vi "acquisition test fixed exposure 6.vi"() -> ()   [LabVIEW 2023]
uses:
  <vilib>/userDefined/High Color/IMAQdx.ctl
  <vilib>/vision/driver/IMAQdx.llb/IMAQdx Acquisition Mode.ctl
  <vilib>/vision/Avi.llb/IMAQ AVI2 Refnum.ctl
  <vilib>/vision/Image Controls.llb/IMAQ Image.ctl
  <vilib>/vision/driver/IMAQdx.llb/IMAQdx Buffer Number Mode.ctl
  <vilib>/DAQmx/write.llb/DAQmx Write (Analog 1D Wfm NChan NSamp).vi
  <vilib>/DAQmx/read.llb/DAQmx Read (Analog 1D Wfm NChan NSamp).vi
  <extravilib>/ChannelInstances/Tag-bool/Read With Abort.vi
  <vilib>/Utility/High Resolution Relative Seconds.vi
  <extravilib>/ChannelInstances/Tag-bool/Write With Abort.vi
  <vilib>/DAQmx/create/channels.llb/DAQmx Create Channel (AI-Voltage-Basic).vi
  <vilib>/DAQmx/configure/timing.llb/DAQmx Timing (Sample Clock).vi
  <vilib>/DAQmx/create/channels.llb/DAQmx Create Channel (AO-Voltage-Basic).vi
  <vilib>/DAQmx/configure/trigger.llb/DAQmx Start Trigger (Digital Edge).vi
  <vilib>/DAQmx/miscellaneous.llb/DAQmx Fill In Error Info.vi
  <extravilib>/ChannelInstances/Tag-bool/Instantiate.vi
  <extravilib>/ChannelInstances/Tag-bool/EndpointRead.vi
  <vilib>/vision/EDVR.llb/IMAQ ImageToEDVR.vi
  <vilib>/vision/EDVR.llb/IMAQ ImageToEDVR 1D U8.vi
  <vilib>/vision/EDVR.llb/IMAQ ImageToEDVR 1D I16.vi
  <vilib>/vision/EDVR.llb/IMAQ ImageToEDVR 1D U32.vi
  <vilib>/vision/EDVR.llb/IMAQ ImageToEDVR 1D U16.vi
  <vilib>/Utility/file.llb/Write Delimited Spreadsheet (string).vi
  <extravilib>/ChannelInstances/Tag-bool/Endpoint.vi
  <vilib>/Waveform/WDTOps.llb/WDT Append Waveforms DBL.vi
  <extravilib>/ChannelInstances/Tag-bool.lvlib
  <vilib>/vision/driver/NI_Vision_Acquisition_Software.lvlib
  <resource>/objmgr/imaqdx.rc
  <vilib>/measure/NI_MABase.lvlib
  <resource>/objmgr/daqmx.rc
panel:
  out "Image Display":T1(plugin-control)
  out "SampClk.Rate":dbl
  in  "stop 2":bool
  out "Waveform Graph":waveform(dbl)[](graph)
  in  "Cluster 5":T2={"Cluster"={"signal type"=enum."Square Wave", "Frequency"=0.0, "Amplitude"=0.0, "Phase"=0.0, "Offset"=0.0, "Duty Cycle"=0.0}, "Cluster 2"={"signal type"=enum."Square Wave", "Frequency"=0.0, "Amplitude"=0.0, "Phase"=0.0, "Offset"=0.0, "Duty Cycle"=0.0}, "Cluster 3"={"signal type"=enum."Square Wave", "Frequency"=0.0, "Amplitude"=0.0, "Phase"=0.0, "Offset"=0.0, "Duty Cycle"=0.0}}
  out "Temp Disk\nSpace (bytes)":i64 format="%.0p"
  out "min until full":dbl
  out "Video Bytes/s":dbl format="%#_3p"
  out "sample\nbytes/s":dbl format="%#_6p"
  out "Sample Rate 3":dbl=100000.0 format="%#_13g"
  out "Delay":dbl
  out "Sample Rate 2":dbl=100000.0 format="%#_13g"
  in  "Update Every n Frames":i32=20
  out "Images Missed":u32
  in  "Camera Control Port":tag="/Dev1/PFI2"
  in  "Exposure Time":dbl=0.0001 format="%#_13g"
  in  "Sample Buffer":i32=100000
  in  "physical channels":tag="Dev1/ai2:3"
  in  "Frame Rate":dbl=150.0 format="%#_13g"
  in  "Sample Rate":dbl=100000.0 format="%#_13g"
  in  "Sync":enum16{"NoSync", "Sync"}(ring)=enum."Sync"
  in  "stop":bool
  in  "File Type":enum16{"AVI", "TDMS", "None"}(ring)
  in  "Codec":u16(ring) items=["No TDMS Codec"]
  out "Image 2":T1(plugin-control)
  in  "Buffer Images":i32=30
  out "Optimizations":T3
  in  "Images per File":i64=10000
  out "Images Behind 2":u32
  out "Write Speed":dbl(graph) caption="Image File Write Speed"
  out "Images Acquired Per Second":dbl
  out "Images Saved Per Second":dbl
  out "Maximum FrameRate":dbl
  out "Sensor Readout Time":dbl
  out "Waveform Chart":waveform(dbl)[](graph)
  in  "stop collection":bool
  # "Y800 for High Framerate\nMotion JPEG for Med-Low"
  # "TDMS Recomended For High Framerate"
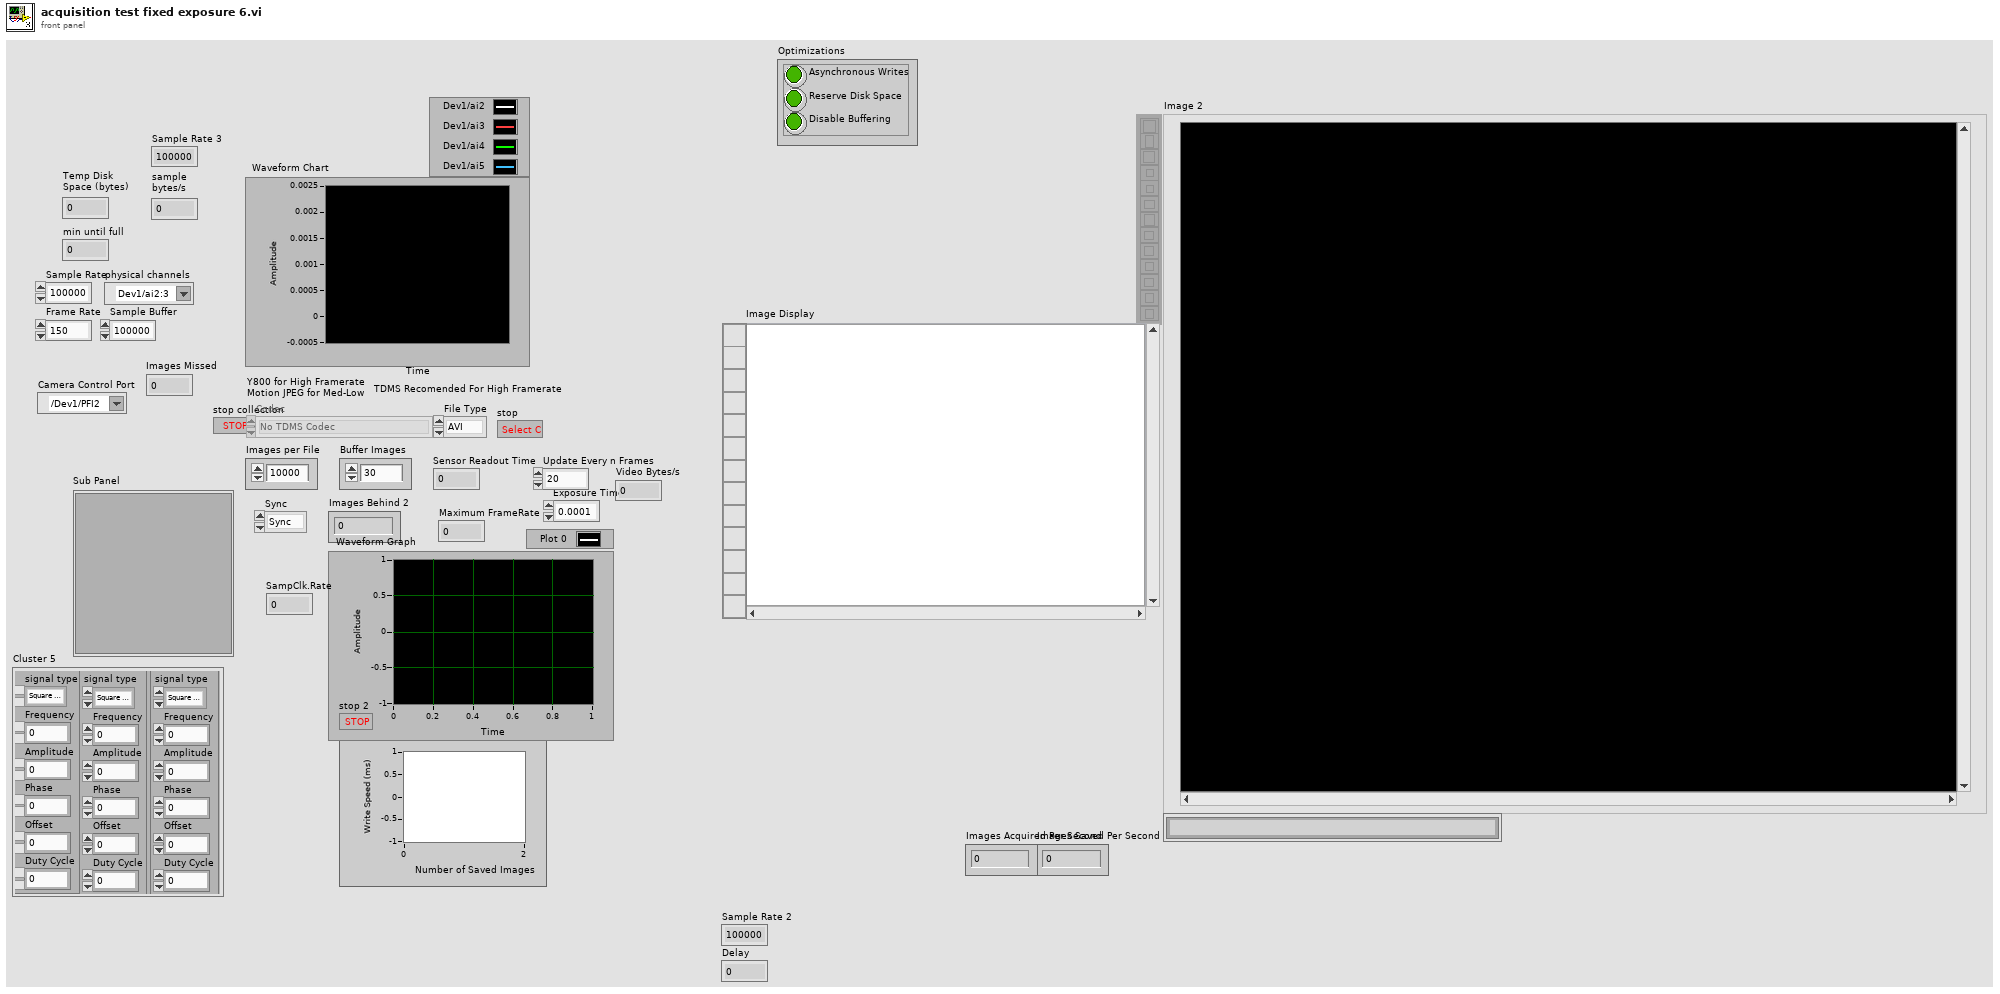
[diagram p1: front panel]
types:
  T1 = typedef "IMAQ Image.ctl" = refnum<image>
  T2 = cluster{"Cluster":cluster{"signal type":enum16{"Sine Wave", "Triangle Wave", "Square Wave", "Sawtooth Wave"}, "Frequency":dbl, "Amplitude":dbl, "Phase":dbl, "Offset":dbl, "Duty Cycle":dbl}, "Cluster 2":cluster{"signal type":enum16{"Sine Wave", "Triangle Wave", "Square Wave", "Sawtooth Wave"}, "Frequency":dbl, "Amplitude":dbl, "Phase":dbl, "Offset":dbl, "Duty Cycle":dbl}, "Cluster 3":cluster{"signal type":enum16{"Sine Wave", "Triangle Wave", "Square Wave", "Sawtooth Wave"}, "Frequency":dbl, "Amplitude":dbl, "Phase":dbl, "Offset":dbl, "Duty Cycle":dbl}}
  T3 = cluster{"Asynchronous Writes":bool, "Reserve Disk Space":bool, "Disable Buffering":bool}
  T4 = enum16{"open", "open or create", "create or replace", "create", "open (read-only)"}
  T5 = cluster{"Images Acquired Per Second":refnum<vi>, "Images Saved Per Second":refnum<vi>, "Images Behind 2":refnum<vi>, "Images Missed":refnum<vi>, "Write Speed":refnum<vi>, " Image Display":refnum<vi>}
  T6 = cluster{"Display N Frames":i32, "File Type":enum16{"AVI", "TDMS", "None"}, "Images Per File":i32, "Quality":i32, "Codec":string, "path":path, "FPS":i32}
  T7 = typedef "Image Type" = u32
  T8 = typedef "IMAQ AVI2 Refnum.ctl" = refnum<k20>
  T9 = cluster{"TDMS Ref":refnum<k34>, "TDMS Write Settings":cluster{"Image Type":T7, "Async File Format":bool}, "AVI Ref":T8}
  T10 = cluster{"Width":u32, "Height":u32, "Format":u32, "Bit Depth":u32}
  T11 = typedef "NI_Vision_Acquisition_Software.lvlib/IMAQdx Acquisition Mode.ctl" = enum32{"One Shot", "Continuous"}
  T12 = enum16{"Exposure End", "Exposure Center", "Exposure Start", "Start", "NoSync"}
  T13 = typedef "IMAQdx.ctl" = refnum<k21>
  T14 = enum8{"Enabled", "Disabled", "Disabled and Grayed Out"}
  T15 = cluster{"Image Type":T7, "Async File Format":bool}
  T16 = cluster{"High Time":dbl, "Low Time":dbl, "Delay":dbl}
  T17 = cluster{"signal type":enum16{"Sine Wave", "Triangle Wave", "Square Wave", "Sawtooth Wave"}, "Frequency":dbl, "Amplitude":dbl, "Phase":dbl, "Offset":dbl, "Duty Cycle":dbl}[]
  T18 = enum16{"Sine Wave", "Triangle Wave", "Square Wave", "Sawtooth Wave"}
  T19 = typedef "Tag-bool.lvlib/))Channel.ctl" = refnum<queue>
  T20 = typedef "NI_Vision_Acquisition_Software.lvlib/IMAQdx Buffer Number Mode.ctl" = enum32{"Next", "Last", "Buffer Number", "Every", "Last New"}
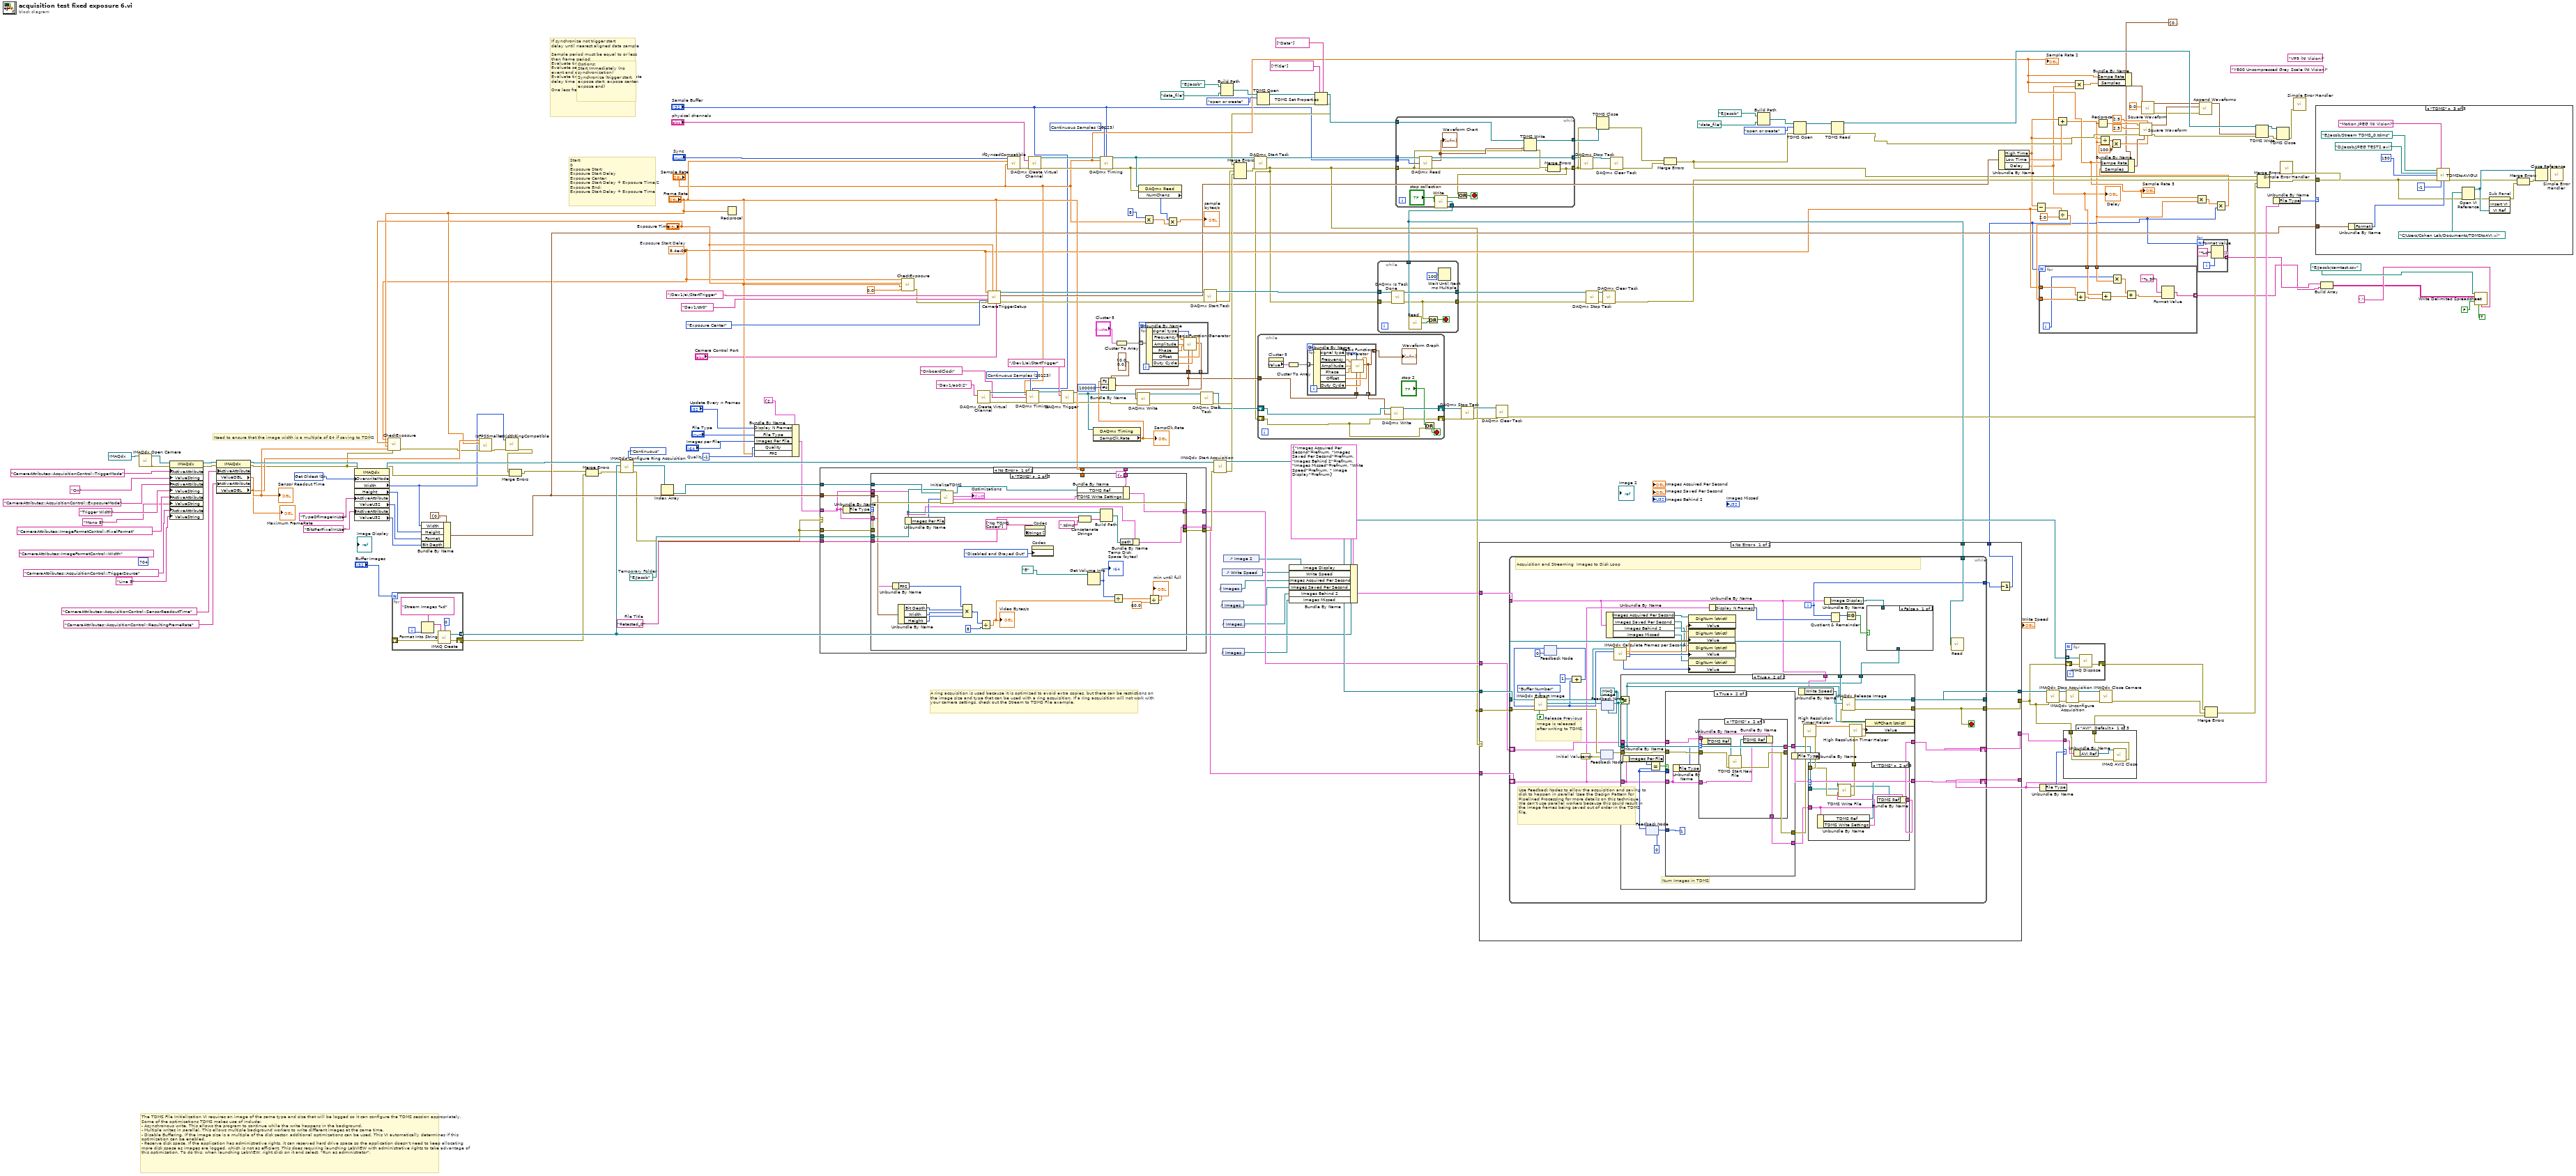
[diagram p0: block diagram]
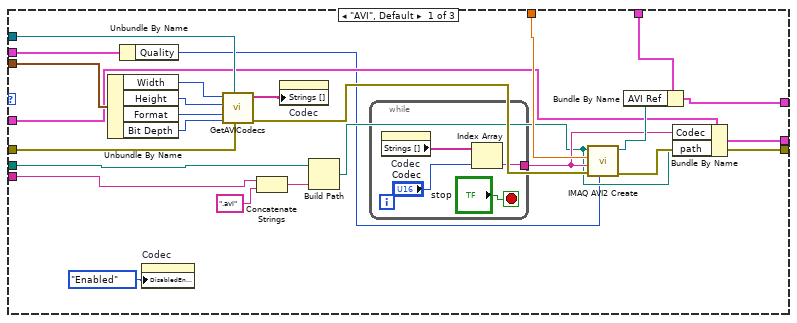
[diagram p4: hidden frame]
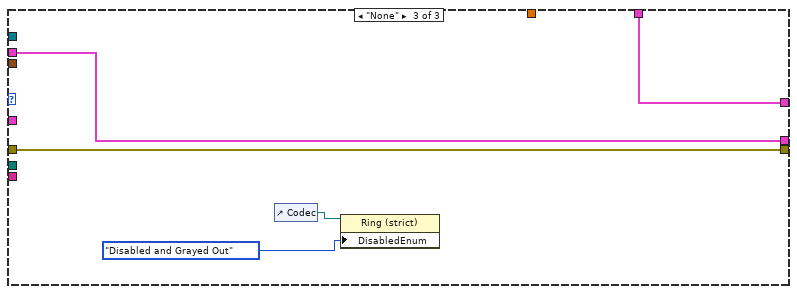
[diagram p5: hidden frame]
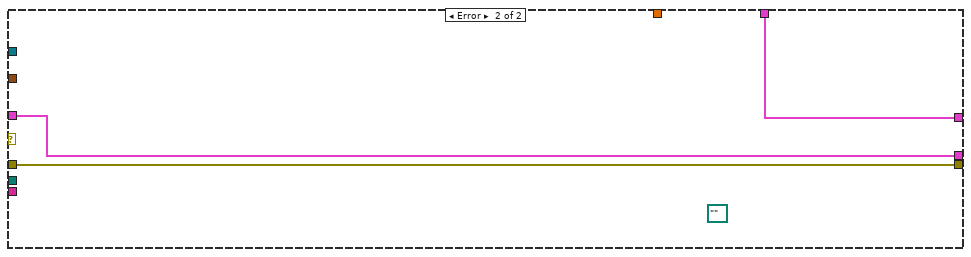
[diagram p6: hidden frame]
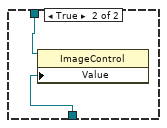
[diagram p7: hidden frame]
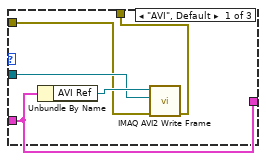
[diagram p9: hidden frame]
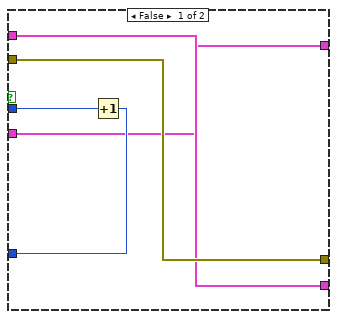
[diagram p11: hidden frame]
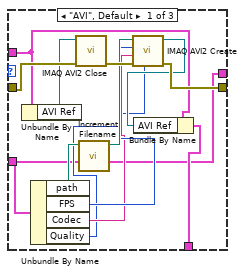
[diagram p12: hidden frame]
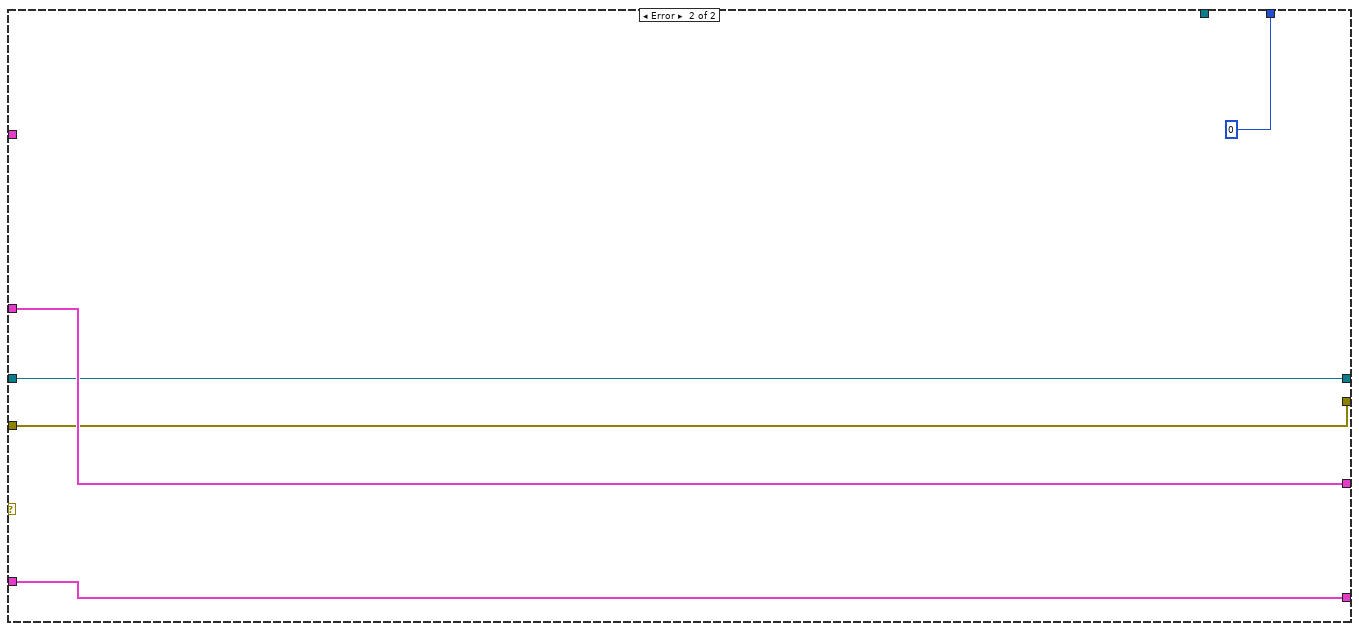
[diagram p14: hidden frame]
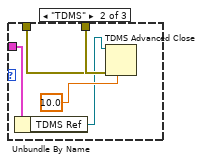
[diagram p15: hidden frame]
diagram:
  (unwired) i64 704 ("ValueI64")
  (unwired) "CameraAttributes::ImageFormatControl::Width" ("ActiveAttribute")
  w47 = 10123 items=["Finite Samples"=10178, "Continuous Samples"=10123, "Hardware Timed Single Point"=12522] ("sample mode")
  w65 = cluster{"Sampe Rate":dbl, "Samples":dbl} {"Sampe Rate"=0.0, "Samples"=0.0}
  w19 = 8.4e-06  # Exposure Start Delay
  w121 = -1  # Quality
  w156 = path "E:/Jacob"  # Temporary Folder
  (unwired) "Y800 Uncompressed Grey Scale (NI Vision)" ("Codec")
  (unwired) "VP9 (NI Vision)" ("Codec")
  w166 = u32 0 items=["Get Oldest"=0, "Fail"=2, "Get Newest"=3] ("OverwriteMode")
  w154 = "Retested_0"  # File Title
  w202 = 10123 items=["Finite Samples"=10178, "Continuous Samples"=10123, "Hardware Timed Single Point"=12522] ("sample mode")
  # "Need to ensure that the image width is a multiple of 64 if saving to TDMS"
  # "The TDMS File Initialization VI requires an image of the same type and size that will be logged so it can configure the TDMS session appropriately. Some of the optimizations TDMS makes use of include:\n- Asynchronous write. This allows the program to continue while the write happens in the background.\n- Multiple writes in parallel. This allows multiple background workers to write different images at the same time.\n- Disable Buffering. If the image size is a multiple of the disk sector, additional optimizations can be used. This VI automatically determines if this optimization can be enabled.\n- Reserve disk space. If the application has administrative rights, it can reserved hard drive space so the application doesn't need to keep allocating more disk space as images are logged, which is not as efficient. This does requiring launching LabVIEW with administrative rights to take advantage of this optimization. To do this, when launching LabVIEW, right click on it and select, \"Run as administrator\"."
  # "A ring acquisition is used because it is optimized to avoid extra copies, but there can be restrictions on the image size and type that can be used with a ring acquisition. If a ring acquisition will not work with your camera settings, check out the Stream to TDMS File example."
  # "Start:\n0\nExposure Start:\nExposure Start Delay\nExposure Center:\nExposure Start Delay + Exposure Time/2\nExposure End:\nExposure Start Delay + Exposure Time"
  # "If synchronize not trigger start\ndelay until nearest aligned data sample\n\nSample period must be equal to or less than frame period\nEvaluate time from pulse until event\nEvaluate samples between pulse and event and extract remainder\nEvaluate time of 1-remainder to calculate delay time\n\nOne less frame than data"
  # "Options:\nStart Immediately (no synchronization)\nSynchronize (trigger start, expose start, expose center, expose end)"
  n1 = call <vilib>:"IMAQdx Open Camera.vi"("Session In"=T13 "cam0") -> ("error out"=w138:errorcluster, "Session Out"=w139:T13)  [unwired: 9 in]
  n2 = property class="IMAQdx"(reference=w139, error in=w138, "ActiveAttribute"="CameraAttributes::AcquisitionControl::TriggerMode", "ValueString"="On", "ActiveAttribute"="CameraAttributes::AcquisitionControl::ExposureMode", "ValueString"="Trigger Width", "ActiveAttribute"="CameraAttributes::ImageFormatControl::PixelFormat", "ValueString"="Mono 8", "ActiveAttribute"="CameraAttributes::AcquisitionControl::TriggerSource", "ValueString"="Line 3") -> (reference out=w195:T13, error out=w194:errorcluster)
  n3 = property class="IMAQdx"(reference=w195, error in=w194, "ActiveAttribute"="CameraAttributes::AcquisitionControl::SensorReadoutTime", "ActiveAttribute"="CameraAttributes::AcquisitionControl::ResultingFrameRate") -> (reference out=w165:T13, error out=w94:errorcluster, "ValueDBL"=w135:dbl, "ValueDBL"=w133:dbl)
  "Sensor Readout Time" <- w135
  "Maximum FrameRate" <- w133
  n4 = property class="IMAQdx"(reference=w165, error in=w94, "OverwriteMode"=w166, "ActiveAttribute"="TypeOfImageInUse", "ActiveAttribute"="BitsPerPixelInUse") -> (reference out=w162:T13, error out=w130:errorcluster, "Width"=w2:u32, "Height"=w148:u32, "ValueU32"=w147:u32, "ValueU32"=w146:u32)
  n5 = call "CheckExposure.vi"("error constant"=w94, "Sensor readout time"=w135, "Frame Rate"="Frame Rate", "Exposure Time"="Exposure Time", "Exposure Start Delay"=w19) -> ("error out"=w132:errorcluster)  [unwired: 6 in]
  n6 = for {
    N: "Buffer Images" -> [_]
    tunnel: [w211] -> w161 mode=indexing
    shift-right: [w210] -> w141
    shift-left: _ -> [w212]
    i -> [w209]
    n7 = Format Into String(format string="Stream Images %d" ("Image Name"), w209) -> (resulting string=w208:string)  [unwired: 2 in, 1 out]
    n8 = call "IMAQ Create"("Border Size"=0, "Image Name"=w208, "error in (no error)"=w212) -> ("New Image"=w211:T1, "error out"=w210:errorcluster)  [unwired: 1 in, 1 out]
  }
  n9 = Bundle By Name(cluster=T10 {"Width"=0, "Height"=0, "Format"=0, "Bit Depth"=0} ("input cluster"), "Width"=w2, "Height"=w148, "Format"=w147, "Bit Depth"=w146) -> (w142:T10)
  n10 = call "IsFPSSmaller.vi"("error constant"=w132, "Frame Rate"="Frame Rate", "Max FrameRate"=w133) -> ("error out"=w131:errorcluster)  [unwired: 8 in]
  n11 = call "IsWidthRingCompatible.vi"("error in (no error)"=w131, "Width"=w2) -> ("error out"=w129:errorcluster)  [unwired: 9 in]
  n12 = Merge Errors(w129, w130) -> (w128:errorcluster)
  n13 = Merge Errors(w128, w141) -> (w140:errorcluster)
  n14 = call <vilib>:"IMAQdx Configure Ring Acquisition.vi"("Mode"=IMAQdx_Acquisition_Mode."Continuous" ("Continuous?"), "error in"=w140, "Images"=w161, "Session In"=w162) -> ("error out"=w127:errorcluster, "Images Out"=w169:T1[], "Session Out"=w173:T13)  [unwired: 5 in]
  n15 = Index Array(array=w169) -> (element=w168:T1)  [unwired: 1 in]
  n16 = Reciprocal(x="Frame Rate") -> ()  [unwired: 1 out]
  n17 = Bundle By Name(cluster=T6 {"Display N Frames"=20, "File Type"=enum."None", "Images Per File"=1000, "Quality"=0, "Codec"="", "path"=path "", "FPS"=0}, "Display N Frames"="Update Every n Frames", "File Type"="File Type", "Images Per File"="Images per File", "Quality"=w121, "FPS"="Frame Rate") -> (w120:T6)
  n18 = case shown="No Error" w127 {
    tunnel: w168 -> [w224 _]
    tunnel: [w223 w292] -> w167
    tunnel: w127 -> [w222 w292]
    tunnel: w156 -> [w221 _]
    tunnel: w154 -> [w220 _]
    tunnel: T9 {"TDMS Ref"=refnum, "TDMS Write Settings"={"Image Type"=0, "Async File Format"=FALSE}, "AVI Ref"=refnum} -> [w219 w293]
    tunnel: [w218 w293] -> w144
    tunnel: w142 -> [w217 _]
    tunnel: "Frame Rate" -> [w216 _]
    tunnel: w120 -> [w213 w291]
    tunnel: [w214 w291] -> w119
    frame No Error {
      n19 = Unbundle By Name(w213) -> ("File Type"=w215:enum16{"AVI", "TDMS", "None"})
      n20 = case shown="\"TDMS\"" w215 {
        tunnel: w224 -> [w237 w285 _]
        tunnel: [w235 w284 w289] -> w223
        tunnel: w222 -> [w245 w283 w289]
        tunnel: w221 -> [w238 w277 _]
        tunnel: w220 -> [w241 w278 _]
        tunnel: w217 -> [w249 w267 _]
        tunnel: w216 -> [w242 _ _]
        tunnel: w219 -> [w234 w275 w288]
        tunnel: [w232 w274 w288] -> w218
        tunnel: w213 -> [w230 w266 _]
        tunnel: w213 -> [w227 w268 w290]
        tunnel: [w225 w269 w290] -> w214
        frame "AVI", Default {
          n21 = Unbundle By Name(w249) -> ("Width"=w236:u32, "Height"=w248:u32, "Format"=w247:u32, "Bit Depth"=w246:u32)
          n22 = Unbundle By Name(w227) -> ("Quality"=w226:i32)
          n23 = property on="Codec" class="Ring (strict)"("DisabledEnum"=T14."Enabled" ("Disabled")) -> ()  [unwired: 2 in, 2 out]
          n24 = call "GetAVICodecs.vi"("error in (no error)"=w245, "Refnum in"=w237, "Bit Depth"=w246, "Format"=w247, "Height"=w248, "Width"=w236) -> ("error out"=w243:errorcluster, "Codec Names"=w244:string[])  [unwired: 4 in]
          n25 = Concatenate Strings(w241, ".avi" ("string")) -> (w239:string)
          n26 = property on="Codec" class="Ring (strict)"("Strings []"=w244) -> ()  [unwired: 2 in, 2 out]
          n27 = Build Path(base path=w238, name or relative path=w239) -> (appended path=w228:path)
          n28 = while {
            tunnel: [w251] -> w229
            stop <- "stop" stop-if-true
            n29 = property on="Codec" class="Ring (strict)"() -> ("Strings []"=w253:string[])  [unwired: 2 in, 2 out]
            n30 = Index Array(array=w253, index="Codec") -> (element=w251:string)
          }
          n31 = call "IMAQ AVI2 Create"("Quality"=w226, "error in (no error)"=w243, "Codec"=w229, "Frames Per Second"=w242, "AVI Path"=w228) -> ("error out"=w235:errorcluster, "AVI Refnum"=w233:T8)  [unwired: 5 in]
          n32 = Bundle By Name(cluster=w234, "AVI Ref"=w233) -> (w232:T9)
          n33 = Bundle By Name(cluster=w230, "Codec"=w229, "path"=w228) -> (w225:T6)
        }
        frame "TDMS" {
          n34 = Unbundle By Name(w266) -> ("FPS"=w262:i32)
          n35 = Unbundle By Name(w267) -> ("Bit Depth"=w263:u32, "Width"=w264:u32, "Height"=w265:u32)
          n36 = Unbundle By Name(w268) -> ("Images Per File"=w271:i32)
          n37 = call "InitializeTDMS.vi"("FilePath"=w277, "error in (no error)"=w283, "Images per File"=w271, "Image Ref in"=w285) -> ("error out"=w284:errorcluster, "Write Settings Out"=w272:T15, "Optimizations"=→"Optimizations":T3, "Refnum out"=w273:refnum<k34>)  [unwired: 4 in]
          n38 = Compound Arithmetic op=MULTIPLY(w262, w263, w264, w265) -> (w261:u32)
          n39 = Divide(x=w261, y=u32 8) -> (x/y=w258:dbl)
          "Video Bytes/s" <- w258
          n40 = property on="Codec" class="Ring (strict)"("Strings []"=string[] ["No TDMS Codec"]) -> ()  [unwired: 2 in, 2 out]
          n41 = property on="Codec" class="Ring (strict)"("DisabledEnum"=T14."Disabled and Grayed Out" ("Disabled")) -> ()  [unwired: 2 in, 2 out]
          n42 = Bundle By Name(cluster=w275, "TDMS Ref"=w273, "TDMS Write Settings"=w272) -> (w274:T9)
          n43 = Concatenate Strings(w278, ".tdms" ("string")) -> (w276:string)
          n44 = Get Volume Info(11:path "E:/" ("path")) -> (1:w254:i64)  [unwired: 1 in, 5 out]
          "Temp Disk\nSpace (bytes)" <- w254
          n45 = Build Path(base path=w277, name or relative path=w276) -> (appended path=w270:path)
          n46 = Divide(x=w254, y=w258) -> (x/y=w257:dbl)
          n47 = Bundle By Name(cluster=w268, "path"=w270) -> (w269:T6)
          n48 = Divide(x=w257, y=60.0) -> (x/y=→"min until full":dbl)
        }
        frame "None" {
          n49 = control-ref of="Codec"() -> (w287:refnum<vi>)
          n50 = property on="Property Node" class="Ring (strict)"(reference=w287, "DisabledEnum"=T14."Disabled and Grayed Out" ("Disabled")) -> ()  [unwired: 1 in, 2 out]
        }
      }
    }
    frame Error {
      (unwired) path "" ("appended path")
    }
  }
  n51 = call "CheckExposure.vi"("Sensor readout time"=0.0, "Frame Rate"="Frame Rate", "Exposure Time"="Exposure Time", "Exposure Start Delay"=w19) -> ("error out"=w136:errorcluster)  [unwired: 7 in]
  n52 = call-poly <vilib>:"DAQmx Create Virtual Channel.vi"("physical channels"=tag "Dev1/ao0:2") -> ("task out"=w48:refnum<k21>, "error out"=w49:errorcluster)  [unwired: 13 in]
  n53 = call "CameraTriggerSetup.vi"("Camera\nTrigger\nOutput"="Camera Control Port", "Frame Rate"="Frame Rate", "Sync Type"=T12."Exposure Center", "Exposure Time"="Exposure Time", "error in"=w136, "Camera\nClock\nCounter"=tag "Dev1/ctr0" ("counter"), "Start Trigger Source"=tag "/Dev1/ai/StartTrigger" ("source"), "Exposure Start Delay"=w19) -> ("error out"=w72:errorcluster, "CameraSignalDefinition"=w87:T16, "CameraSignalRefnum"=w184:refnum<k21>)  [unwired: 1 in]
  n54 = call "IfSyncedCompatible.vi"("Sample Rate"="Sample Rate", "Frame Rate"="Frame Rate", "Enum"="Sync") -> ("error out"=w152:errorcluster)  [unwired: 8 in]
  n55 = call-poly <vilib>:"DAQmx Timing.vi"("task/channels in"=w48, "sample mode"=w47, "samples per channel"="Sample Buffer", "rate"="Sample Rate", "source"=tag "OnboardClock", "error in"=w49) -> ("task out"=w45:refnum<k21>, "error out"=w44:errorcluster)  [unwired: 8 in]
  n56 = call-poly <vilib>:"DAQmx Create Virtual Channel.vi"("physical channels"="physical channels", "error in"=w152) -> ("task out"=w205:refnum<k21>, "error out"=w204:errorcluster)  [unwired: 12 in]
  n57 = call-poly <vilib>:"DAQmx Trigger.vi"("task/channels in"=w45, "source"=tag "/Dev1/ai/StartTrigger", "error in"=w44) -> ("task out"=w36:refnum<k21>, "error out"=w39:errorcluster)  [unwired: 11 in]
  n58 = property class="DAQmx Timing"(reference=w36) -> ("SampClk.Rate"=w28:dbl)  [unwired: 1 in, 2 out]
  "SampClk.Rate" <- w28
  n59 = call-poly <vilib>:"DAQmx Timing.vi"("task/channels in"=w205, "sample mode"=w202, "samples per channel"="Sample Buffer", "rate"="Sample Rate", "error in"=w204) -> ("task out"=w56:refnum<k21>, "error out"=w55:errorcluster)  [unwired: 9 in]
  n60 = Bundle By Name(cluster=cluster{"Fs":dbl, "#s":dbl} {"Fs"=0.0, "#s"=0.0} ("sampling info"), "Fs"=w28, "#s"=100000) -> (w26:cluster{"Fs":dbl, "#s":dbl})
  n61 = Cluster To Array(cluster="Cluster 5") -> (array=w41:T17)
  n62 = property class="DAQmx Read"(reference=w56, error in=w55) -> ("NumChans"=w52:u32)  [unwired: 2 out]
  n63 = for {
    tunnel: w41 -> [w302] mode=indexing
    tunnel: [w296] -> w40 mode=indexing
    tunnel: w26 -> [w295]
    n64 = Unbundle By Name(w302) -> ("signal type"=w294:T18, "Frequency"=w301:dbl, "Amplitude"=w300:dbl, "Phase"=w299:dbl, "Offset"=w298:dbl, "Duty Cycle"=w297:dbl)
    n65 = call <vilib>:"Basic Function Generator.vi"("offset"=w298, "square wave duty cycle (%)"=w297, "sampling info"=w295, "signal type"=w294, "phase"=w299, "amplitude"=w300, "frequency"=w301) -> ("signal out"=w296:waveform(dbl))  [unwired: 2 in, 2 out]
  }
  n66 = call-poly <vilib>:"DAQmx Write.vi"("task/channels in"=w36, "data"=w40, "error in"=w39) -> ("task out"=w38:refnum<k21>, "error out"=w37:errorcluster)  [unwired: 10 in, 1 out]
  n67 = Multiply(x=8, y="Sample Rate") -> (x*y=w53:dbl)
  n68 = Multiply(x=w52, y=w53) -> (x*y=→"sample\nbytes/s":dbl)
  n69 = call <vilib>:"DAQmx Start Task.vi"("task/channels in"=w38, "error in"=w37) -> ("task out"=w33:refnum<k21>, "error out"=w34:errorcluster)  [unwired: 12 in]
  n70 = call <vilib>:"DAQmx Start Task.vi"("task/channels in"=w184, "error in"=w72) -> ("task out"=w183:refnum<k21>, "error out"=w180:errorcluster)  [unwired: 12 in]
  n71 = call <vilib>:"IMAQdx Start Acquisition.vi"("error in"=w167, "Session In"=w173) -> ("error out"=w163:errorcluster, "Session Out"=w170:T13)  [unwired: 8 out]
  n72 = control-ref of="Images Acquired Per Second"() -> (w111:refnum<vi>)
  n73 = Build Path(base path=path "E:/Jacob", name or relative path=path "data_file") -> (appended path=w105:path)
  n74 = control-ref of="Images Saved Per Second"() -> (w110:refnum<vi>)
  n75 = control-ref of="Write Speed"() -> (w115:refnum<vi>)
  n76 = control-ref of="Images Missed"() -> (w108:refnum<vi>)
  n77 = control-ref of="Image 2"() -> (w116:refnum<vi>)
  n78 = control-ref of="Images Behind 2"() -> (w109:refnum<vi>)
  n79 = TDMS Open(10:T4."open or create" ("operation (0:open)"), 11:w105) -> (0:w107:errorcluster, 3:w106:refnum<k34>)  [unwired: 5 in]
  n80 = Bundle By Name(cluster=T5 {"Images Acquired Per Second"=refnum, "Images Saved Per Second"=refnum, "Images Behind 2"=refnum, "Images Missed"=refnum, "Write Speed"=refnum, " Image Display"=refnum}, "Image Display"=w116, "Write Speed"=w115, "Images Acquired Per Second"=w111, "Images Saved Per Second"=w110, "Images Behind 2"=w109, "Images Missed"=w108) -> (w114:T5)
  n81 = TDMS Set Properties(5:string[] ["Data"] ("property values"), 7:string[] ["Title"] ("property names"), 8:w107, 11:w106) -> (0:w8:errorcluster, 3:w102:refnum<k34>)  [unwired: 2 in, 2 out]
  n82 = Merge Errors(w8, w55, w180, w163, w34) -> (w181:errorcluster)
  n83 = call <vilib>:"DAQmx Start Task.vi"("task/channels in"=w56, "error in"=w181) -> ("task out"=w182:refnum<k21>, "error out"=w7:errorcluster)  [unwired: 12 in]
  n84 = while {
    tunnel: w26 -> [w311]
    shift-right: [w310] -> w32
    shift-left: w33 -> [w309]
    shift-right: [w305] -> w31
    shift-left: w7 -> [w303]
    stop <- w304 stop-if-true
    n85 = property on="Cluster 5" class="Clust (strict)"() -> ("Value"=w313:T2)  [unwired: 2 in, 2 out]
    n86 = Cluster To Array(cluster=w313) -> (array=w312:T17)
    n87 = for {
      tunnel: w312 -> [w322] mode=indexing
      tunnel: [w314] -> w308 mode=indexing
      tunnel: w311 -> [w315]
      tunnel: [w314] -> w307 mode=indexing
      n88 = Unbundle By Name(w322) -> ("signal type"=w321:T18, "Frequency"=w320:dbl, "Amplitude"=w319:dbl, "Phase"=w318:dbl, "Offset"=w317:dbl, "Duty Cycle"=w316:dbl)
      n89 = call <vilib>:"Basic Function Generator.vi"("offset"=w317, "square wave duty cycle (%)"=w316, "sampling info"=w315, "signal type"=w321, "phase"=w318, "amplitude"=w319, "frequency"=w320) -> ("signal out"=w314:waveform(dbl))  [unwired: 2 in, 2 out]
    }
    "Waveform Graph" <- w307
    n90 = call-poly <vilib>:"DAQmx Write.vi"("task/channels in"=w309, "data"=w308, "error in"=w303) -> ("task out"=w310:refnum<k21>, "error out"=w305:errorcluster)  [unwired: 10 in, 1 out]
    n91 = Or(x="stop 2", y=w303) -> (x .or. y?=w304:bool)
  }
  n92 = while {
    tunnel: [w335] -> w192
    tunnel: [w324] -> w98
    tunnel: w182 -> [w334]
    tunnel: w7 -> [w327]
    tunnel: "Sample Buffer" -> [w333]
    tunnel: [w332] -> w68
    tunnel: w102 -> [w329]
    tunnel: [w323] -> w99
    stop <- w331 stop-if-true
    n93 = call-poly <vilib>:"DAQmx Read.vi"("task/channels in"=w334, "number of samples per channel"=w333, "error in"=w327) -> ("task out"=w335:refnum<k21>, "data"=w328:waveform(dbl)[], "error out"=w325:errorcluster)  [unwired: 10 in]
    "Waveform Chart" <- w328
    n94 = call <extravilib>:"Write.vi"("element"="stop collection") -> ("channel"=w332:T19)  [unwired: 1 out]
    n95 = TDMS Write(0:w329, 9:w328, 11:w327) -> (4:w323:refnum<k34>, 15:w326:errorcluster)  [unwired: 3 in, 2 out]
    n96 = Merge Errors(w326, w325) -> (w324:errorcluster)
    n97 = Or(x=w324, y="stop collection") -> (x .or. y?=w331:bool)
  }
  n98 = while {
    tunnel: w68 -> [w339]
    tunnel: w183 -> [w343]
    tunnel: w7 -> [w342]
    tunnel: [w341] -> w189
    tunnel: [w338] -> w188
    stop <- w336 stop-if-true
    n99 = call <vilib>:"DAQmx Is Task Done.vi"("task/channels in"=w343, "error in"=w342) -> ("task out"=w341:refnum<k21>, "error out"=w338:errorcluster)  [unwired: 11 in, 1 out]
    n100 = call <extravilib>:"Read.vi"("channel"=w339) -> ("element"=w337:bool)  [unwired: 1 in, 1 out]
    n101 = Or(x=w338, y=w337) -> (x .or. y?=w336:bool)
    n102 = Wait Until Next ms Multiple(millisecond multiple=u32 100) -> ()  [unwired: 1 out]
  }
  n103 = call <vilib>:"DAQmx Stop Task.vi"("task/channels in"=w32, "error in"=w31) -> ("task out"=w30:refnum<k21>, "error out"=w29:errorcluster)  [unwired: 12 in]
  n104 = case shown="No Error" w7 {
    tunnel: [w355 w479] -> w171
    tunnel: w170 -> [w354 w479]
    tunnel: w7 -> [w353 w480]
    tunnel: [w352 w480] -> w157
    tunnel: w144 -> [w351 w481]
    tunnel: [w350 w481] -> w143
    tunnel: w119 -> [w349 w478]
    tunnel: [w348 w478] -> w113
    tunnel: w114 -> [w347 _]
    tunnel: w68 -> [w346 _]
    tunnel: [w344 0] -> w16
    frame No Error {
      n105 = while {
        tunnel: w353 -> [w394]
        tunnel: w354 -> [w392]
        tunnel: [w393] -> w355
        tunnel: [w356] -> w352
        shift-right: [w372] -> w350
        shift-left: w351 -> [w373]
        shift-right: [w371] -> w348
        shift-left: w349 -> [w370]
        tunnel: w347 -> [w363]
        tunnel: w346 -> [w358]
        tunnel: [w357] -> w345
        i -> [w357]
        stop <- w356 stop-if-true
        w377 = errorcluster {"status"=FALSE, "code"=0, "source"=""}  # Initial Value
        w390 = FALSE  # Release Previous
        w386 = T1 refnum ("Image Out")
        # "Use Feedback Nodes to allow the acquisition and saving to disk to happen in parallel (see the Design Pattern for Pipelined Processing for more details on this technique). We can't use parallel workers because this could result in the image frames being saved out of order in the TDMS file."
        # "Image is released after writing to TDMS."
        # "Acquisition and Streaming  Images to Disk Loop"
        n106 = feedback #1(u32 0) -> (w379:u32)
        n107 = call <vilib>:"IMAQdx Extract Image.vi"("Release Previous (true)"=w390, "Buffer Number Mode (Next)"=IMAQdx_Buffer_Number_Mode."Buffer Number" ("Buffer Number Mode"), "error in"=w394, "Buffer Number In"=w379, "Session In"=w392) -> ("error out"=w383:errorcluster, "Buffer Number Out"=w381:u32, "Image Out"=w388:T1, "Session Out"=w389:T13)  [unwired: 3 in]
        n108 = Compound Arithmetic op=ADD(u32 1 ("value"), w381) -> (w382:u32)
        n109 = feedback-in #1(w382) -> ()
        n110 = feedback-in #2(w383) -> ()
        n111 = feedback #2(w377) -> (w387:errorcluster)
        n112 = feedback-in #3(w388) -> ()
        n113 = feedback #3(w386) -> (w384:T1)
        n114 = Unbundle By Name(w363) -> ("Images Acquired Per Second"=w362:refnum<vi>, "Images Saved Per Second"=w361:refnum<vi>, "Images Behind 2"=w360:refnum<vi>, "Images Missed"=w359:refnum<vi>)
        n115 = call <vilib>:"IMAQdx Calculate Frames per Second.vi"("Session In"=w389, "Buffer Number"=w381) -> ("Acquired Frames per Second"=w364:dbl, "Processed Frames per Second"=w365:dbl, "Images Behind"=w366:i32, "Images Missed"=w367:u32)  [unwired: 7 in, 3 out]
        n116 = Not Equal?(x=w386, y=w384) -> (x != y?=w385:bool)
        n117 = case shown="True" w385 {
          tunnel: w384 -> [w400 w412]
          tunnel: w387 -> [w397 w421]
          tunnel: [w401 w425] -> w393
          tunnel: w392 -> [w401 w424]
          tunnel: [w397 w423] -> w356
          tunnel: [w400 w412] -> w374
          tunnel: w373 -> [w399 w411]
          tunnel: [w399 w410] -> w372
          tunnel: w370 -> [w398 w406]
          tunnel: [w398 w408] -> w371
          tunnel: w363 -> [_ w403]
          frame False {
            # "First iteration doesn't have valid image for this pipelined stage."
          }
          frame True {
            # "Num Images in TDMS"
            n118 = Unbundle By Name(w406) -> ("Images Per File"=w405:i32)
            n119 = feedback #4(i64 0) -> (w419:i64)
            n120 = Equal?(x=w405, y=w419) -> (x = y?=w420:bool)
            n121 = case shown="True" w420 {
              tunnel: [w445 i64 1] -> w418
              tunnel: w421 -> [w444 w451]
              tunnel: [w444 w452] -> w417
              tunnel: w419 -> [w443 _]
              tunnel: w411 -> [w442 w450]
              tunnel: [w442 w449] -> w409
              tunnel: w406 -> [w441 w447]
              tunnel: [w441 w448] -> w408
              frame False {
                n122 = Increment(x=w443) -> (x+1=w445:i64)
              }
              frame True {
                n123 = Unbundle By Name(w447) -> ("File Type"=w446:enum16{"AVI", "TDMS", "None"})
                n124 = case shown="\"TDMS\"" w446 {
                  tunnel: [w464 w473 w474] -> w452
                  tunnel: w451 -> [w465 w472 w474]
                  tunnel: w450 -> [w462 w470 w476]
                  tunnel: [w460 w468 w476] -> w449
                  tunnel: w447 -> [w454 w467 w475]
                  tunnel: [w454 w467 w475] -> w448
                  frame "AVI", Default {
                    n125 = Unbundle By Name(w462) -> ("AVI Ref"=w463:T8)
                    n126 = Unbundle By Name(w454) -> ("path"=w458:path, "FPS"=w457:i32, "Codec"=w456:string, "Quality"=w455:i32)
                    n127 = call "IMAQ AVI2 Close"("error in (no error)"=w465, "AVI Refnum"=w463) -> ("error out"=w466:errorcluster)  [unwired: 9 in]
                    n128 = call "Increment Filename.vi"("Path In"=w458) -> ("Incremented Path Out"=w459:path)  [unwired: 10 in]
                    n129 = call "IMAQ AVI2 Create"("Quality"=w455, "error in (no error)"=w466, "Codec"=w456, "Frames Per Second"=w457, "AVI Path"=w459) -> ("error out"=w464:errorcluster, "AVI Refnum"=w461:T8)  [unwired: 5 in]
                    n130 = Bundle By Name(cluster=w462, "AVI Ref"=w461) -> (w460:T9)
                  }
                  frame "TDMS" {
                    n131 = Unbundle By Name(w470) -> ("TDMS Ref"=w471:refnum<k34>)
                    n132 = call "TDMS Start New File.vi"("error in"=w472, "Previous TDMS Refnum In"=w471) -> ("error out"=w473:errorcluster, "New TDMS Refnum Out"=w469:refnum<k34>)  [unwired: 8 in]
                    n133 = Bundle By Name(cluster=w470, "TDMS Ref"=w469) -> (w468:T9)
                  }
                  frame "None" {
                  }
                }
              }
            }
            n134 = feedback-in #4(w418) -> ()
            n135 = Unbundle By Name(w408) -> ("File Type"=w407:enum16{"AVI", "TDMS", "None"})
            n136 = Unbundle By Name(w403) -> ("Write Speed"=w402:refnum<vi>)
            n137 = call "High Resolution Timer Helper.vi"("error in (no error)"=w417) -> ("error out"=w416:errorcluster, "Current Time"=w414:dbl)  [unwired: 8 in, 1 out]
            n138 = case shown="\"TDMS\"" w407 {
              tunnel: w416 -> [w428 w438 w439]
              tunnel: [w427 w437 w439] -> w415
              tunnel: w412 -> [w429 w436 _]
              tunnel: w409 -> [w426 w433 w440]
              tunnel: [w426 w431 w440] -> w410
              frame "AVI", Default {
                n139 = Unbundle By Name(w426) -> ("AVI Ref"=w430:T8)
                n140 = call "IMAQ AVI2 Write Frame"("error in (no error)"=w428, "Image"=w429, "AVI Refnum"=w430) -> ("error out"=w427:errorcluster)  [unwired: 6 in, 2 out]
              }
              frame "TDMS" {
                n141 = Unbundle By Name(w433) -> ("TDMS Ref"=w435:refnum<k34>, "TDMS Write Settings"=w434:T15)
                n142 = call "TDMS Write File.vi"("error in"=w438, "Write Settings"=w434, "Image"=w436, "TDMS Ref In"=w435) -> ("error out"=w437:errorcluster, "TDMS Ref Out"=w432:refnum<k34>)  [unwired: 6 in]
                n143 = Bundle By Name(cluster=w433, "TDMS Ref"=w432) -> (w431:T9)
              }
              frame "None" {
              }
            }
            n144 = call "High Resolution Timer Helper.vi"("error in (no error)"=w415, "Previous Time"=w414) -> ("error out"=w413:errorcluster, "Time Difference (ms)"=w404:dbl)  [unwired: 7 in, 1 out]
            n145 = call <vilib>:"IMAQdx Release Image.vi"("error in"=w413, "Image"=w412, "Session In"=w424) -> ("error out"=w423:errorcluster, "Session Out"=w425:T13)  [unwired: 7 in]
            n146 = property on="Property Node" class="WFChart (strict)"(reference=w402, "Value"=w404) -> ()  [unwired: 1 in, 2 out]
          }
        }
        n147 = property on="Property Node" class="DigNum (strict)"(reference=w361, "Value"=w365) -> ()  [unwired: 1 in, 2 out]
        n148 = property on="Property Node" class="DigNum (strict)"(reference=w359, "Value"=w367) -> ()  [unwired: 1 in, 2 out]
        n149 = property on="Property Node" class="DigNum (strict)"(reference=w362, "Value"=w364) -> ()  [unwired: 1 in, 2 out]
        n150 = property on="Property Node" class="DigNum (strict)"(reference=w360, "Value"=w366) -> ()  [unwired: 1 in, 2 out]
        n151 = Unbundle By Name(w370) -> ("Display N Frames"=w369:i32)
        n152 = Unbundle By Name(w363) -> ("Image Display"=w368:refnum<vi>)
        n153 = Quotient & Remainder(x=w357, y=w369) -> (x-y*floor(x/y)=w376:i32)  [unwired: 1 out]
        n154 = Equal To 0?(x=w376) -> (x = 0?=w375:bool)
        n155 = case shown="False" w375 {
          tunnel: w374 -> [_ w395]
          tunnel: w368 -> [_ w396]
          frame False {
          }
          frame True {
            n156 = property on="Property Node" class="ImageControl"(reference=w396, "Value"=w395) -> ()  [unwired: 1 in, 2 out]
          }
        }
        n157 = call <extravilib>:"Read.vi"("channel"=w358) -> ()  [unwired: 1 in, 2 out]
      }
      n158 = Decrement(x=w345) -> (x-1=w344:i32)
    }
    frame Error {
    }
  }
  n159 = call <vilib>:"DAQmx Clear Task.vi"("task in"=w30, "error in"=w29) -> ("error out"=w24:errorcluster)  [unwired: 13 in]
  n160 = call <vilib>:"DAQmx Stop Task.vi"("task/channels in"=w192, "error in"=w98) -> ("task out"=w191:refnum<k21>, "error out"=w179:errorcluster)  [unwired: 12 in]
  n161 = call <vilib>:"DAQmx Stop Task.vi"("task/channels in"=w189, "error in"=w188) -> ("task out"=w193:refnum<k21>, "error out"=w178:errorcluster)  [unwired: 12 in]
  n162 = TDMS Close(8:w98, 11:w99) -> (0:w101:errorcluster)  [unwired: 1 out]
  n163 = call <vilib>:"DAQmx Clear Task.vi"("task in"=w193, "error in"=w178) -> ("error out"=w71:errorcluster)  [unwired: 13 in]
  n164 = call <vilib>:"DAQmx Clear Task.vi"("task in"=w191, "error in"=w179) -> ("error out"=w100:errorcluster)  [unwired: 13 in]
  n165 = Merge Errors(w101, w100) -> (w86:errorcluster)
  n166 = Build Path(base path=path "E:/Jacob", name or relative path=path "data_file") -> (appended path=w93:path)
  n167 = TDMS Open(8:w86, 10:T4."open or create" ("operation (0:open)"), 11:w93) -> (0:w88:errorcluster, 3:w89:refnum<k34>)  [unwired: 4 in]
  n168 = TDMS Read(0:w89, 11:w88) -> (4:w79:refnum<k34>, 15:w78:errorcluster)  [unwired: 6 in, 4 out]
  n169 = Unbundle By Name(w87) -> ("High Time"=w23:dbl, "Low Time"=w85:dbl, "Delay"=w17:dbl)
  "Delay" <- w17
  n170 = Subtract(x=w23, y=w19) -> (x-y=w22:dbl)
  n171 = Unbundle By Name(w113) -> ("File Type"=w118:enum16{"AVI", "TDMS", "None"})
  n172 = call <vilib>:"IMAQdx Stop Acquisition.vi"("error in"=w157, "Session In"=w171) -> ("error out"=w174:errorcluster, "Session Out"=w175:T13)  [unwired: 8 out]
  n173 = Add(x=w23, y=w85) -> (x+y=w18:dbl)
  n174 = Divide(x=w22, y=2.0) -> (x/y=w20:dbl)
  n175 = for {
    N: w16 -> [_]
    tunnel: w20 -> [w492]
    tunnel: w19 -> [w491]
    tunnel: w18 -> [w488]
    tunnel: w17 -> [w489]
    tunnel: [w482] -> w14 mode=indexing
    i -> [w485]
    n176 = Add(x=w491, y=w492) -> (x+y=w490:dbl)
    n177 = Add(x=w489, y=w490) -> (x+y=w487:dbl)
    n178 = Multiply(x=w485, y=w488) -> (x*y=w486:dbl)
    n179 = Add(x=w486, y=w487) -> (x+y=w484:dbl)
    n180 = Format Value(format string="%.9f", value (0)=w484) -> (output string=w482:string)  [unwired: 1 in]
  }
  n181 = case shown="\"AVI\", Default" w118 {
    tunnel: [w493 w500 w502] -> w160
    tunnel: w157 -> [w494 w499 w502]
    tunnel: w143 -> [w496 w498 _]
    frame "AVI", Default {
      n182 = Unbundle By Name(w496) -> ("AVI Ref"=w495:T8)
      n183 = call "IMAQ AVI2 Close"("error in (no error)"=w494, "AVI Refnum"=w495) -> ("error out"=w493:errorcluster)  [unwired: 9 in]
    }
    frame "TDMS" {
      n184 = Unbundle By Name(w498) -> ("TDMS Ref"=w497:refnum<k34>)
      n185 = TDMS Advanced Close(6:10.0 ("timeout (10 s)"), 8:w499, 11:w497) -> (0:w500:errorcluster)  [unwired: 1 in, 1 out]
    }
    frame "None" {
    }
  }
  n186 = for {
    shift-right: [w504] -> w158
    shift-left: w157 -> [w505]
    tunnel: w161 -> [w503] mode=indexing
    n187 = call "IMAQ Dispose"("Image"=w503, "error in (no error)"=w505) -> ("error out"=w504:errorcluster)  [unwired: 4 in]
  }
  n188 = call <vilib>:"IMAQdx Unconfigure Acquisition.vi"("error in"=w174, "Session In"=w175) -> ("error out"=w177:errorcluster, "Session Out"=w176:T13)  [unwired: 8 out]
  n189 = Multiply(x="Sample Rate", y=w17) -> (x*y=w64:dbl)
  n190 = Reciprocal(x=w18) -> (1/x=w70:dbl)
  n191 = Bundle By Name(cluster=w65, "Sampe Rate"="Sample Rate", "Samples"=w64) -> (w63:cluster{"Sampe Rate":dbl, "Samples":dbl})
  n192 = Divide(x=w23, y=w18) -> (x/y=w84:dbl)
  n193 = call <vilib>:"IMAQdx Close Camera.vi"("error in"=w177, "Session In"=w176) -> ("error out"=w159:errorcluster)  [unwired: 9 out]
  n194 = Multiply(x=w84, y=100.0) -> (x*y=w69:dbl)
  n195 = call <vilib>:"Square Waveform.vi"("sampling info"=w63, "amplitude"=0.0) -> ("error out"=w60:errorcluster, "signal out"=w62:waveform(dbl))  [unwired: 8 in]
  n196 = Multiply(x="Sample Rate", y=w18) -> (x*y=w58:dbl)
  n197 = for {
    N: w16 -> [_]
    tunnel: [w506] -> w15 mode=indexing
    i -> [w508]
    n198 = Format Value(format string="%d", value (0)=w508) -> (output string=w506:string)  [unwired: 1 in]
  }
  n199 = Merge Errors(w158, w159, w160) -> (w155:errorcluster)
  n200 = Multiply(x=w58, y=w16) -> (x*y=w57:dbl)
  n201 = Bundle By Name(cluster=w65, "Sampe Rate"="Sample Rate", "Samples"=w57) -> (w80:cluster{"Sampe Rate":dbl, "Samples":dbl})
  n202 = call <vilib>:"Square Waveform.vi"("duty cycle (%)"=w69, "offset"=2.5, "sampling info"=w80, "error in (no error)"=w78, "amplitude"=2.5, "frequency"=w70) -> ("error out"=w67:errorcluster, "signal out"=w61:waveform(dbl))  [unwired: 4 in]
  n203 = call-poly <vilib>:"Append Waveforms.vi"("error in (no error)"=w60, "waveform B"=w61, "waveform A"=w62) -> ("waveform out"=w59:waveform(dbl))  [unwired: 7 in, 1 out]
  n204 = TDMS Write(0:w79, 9:w59, 11:w67) -> (4:w77:refnum<k34>, 15:w76:errorcluster)  [unwired: 3 in, 2 out]
  n205 = Merge Errors(w86, w71, w155, w24) -> (w126:errorcluster)
  n206 = Unbundle By Name(w113) -> ("File Type"=w112:enum16{"AVI", "TDMS", "None"})
  n207 = TDMS Close(8:w76, 11:w77) -> (0:w75:errorcluster)  [unwired: 1 out]
  n208 = call <vilib>:"Simple Error Handler.vi"("error in (no error)"=w126) -> ()  [unwired: 4 in, 5 out]
  n209 = call <vilib>:"Simple Error Handler.vi"("error in (no error)"=w75) -> ()  [unwired: 4 in, 5 out]
  n210 = case shown="\"TDMS\"" w112 {
    tunnel: w142 -> [_ _ w514]
    tunnel: w126 -> [_ _ w512]
    frame "AVI", Default {
    }
    frame "None" {
    }
    frame "TDMS" {
      n211 = Unbundle By Name(w514) -> ("Format"=w513:u32)
      n212 = call "TDMStoAVIGUI.vi"("TDMS Path"=path "E:/Jacob/Stream TDMS_0.tdms" ("AVI Path"), "Codec"="Motion JPEG (NI Vision)", "AVI Out Path"=path "D:/Jacob/JPEG TEST2.avi" ("AVI Path"), "Frames Per Second"=u32 150, "error in (no error)"=w512, "Quality"=-1, "Image Type"=w513) -> ("error out"=w510:errorcluster)  [unwired: 8 in]
      n213 = Open VI Reference(vi path=path "C:/Users/Cohen Lab/Documents/TDMStoAVI.vi", error in (no error)=w512) -> (vi reference=w520:refnum<vi>, error out=w519:errorcluster)  [unwired: 4 in]
      n214 = invoke on="Sub Panel" class="SubPnl" method="Insert VI"(error in=w519, "VI Ref"=w520) -> (error out=w511:errorcluster)  [unwired: 2 in, 3 out]
      n215 = Merge Errors(w510, w511) -> (w509:errorcluster)
      n216 = Close Reference(reference=w520, error in (no error)=w509) -> ()  [unwired: 1 out]
      n217 = call <vilib>:"Simple Error Handler.vi"() -> ()  [unwired: 5 in, 5 out]
    }
  }
  n218 = Build Array(w15, w14) -> (w9:string[][])
  n219 = call-poly <vilib>:"Write Delimited Spreadsheet.vi"("file path (dialog if empty)"=path "E:/Jacob/camtest.csv", "2D data"=w9, "append to file? (new file:F)"=FALSE, "transpose? (no:F)"=TRUE, "delimiter (\\t)"="," ("delimiter (\\t)")) -> ()  [unwired: 9 in, 2 out]
  "Sample Rate 2" <- "Sample Rate"
  "Sample Rate 3" <- "Sample Rate"
